vi "Last Ack Event.vi"(10 "Event":refnum<class "Event jettl.lvclass">, 11 "Last Ack Event in":refnum<class "Last Ack Event.lvclass">) -> (3 "Last Ack Event out":refnum<class "Last Ack Event.lvclass">)   [LabVIEW 2021, in "jettl.lvlib" / "jettl Msg Last Ack Event.lvlib" / "Last Ack Event.lvclass"]
uses:
  Last Ack Event.lvclass
  Event jettl/Event jettl.lvclass
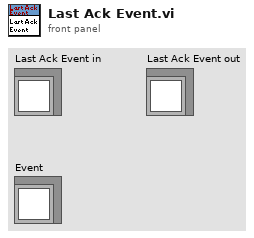
[diagram p1: front panel]
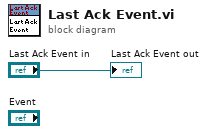
[diagram p0: block diagram]
diagram:
  "Last Ack Event out" <- "Last Ack Event in"
